vi "SetNumber.vi"(6 "i":i32, 7 "Agentes Disponíveis":dbl, 10 "Used numbers":dbl[](array[numeric]), 11 "element":T1={"id"=0, "function"=enum."Attacker", "x"=0.0, "y"=0.0, "orientation"=0.0, "v_tangent"=0.0, "v_normal"=0.0, "v_ang"=0.0, "kick_x"=0.0, "kick_z"=0.0, "dribble"=FALSE, "Timestamp"=timestamp(0 s since 1904-01-01), "estimatives"={"est_v_tangent"=0.0, "est_v_normal"=0.0, "est_vx"=0.0, "est_vy"=0.0, "Pos Robot Est"=[]}, "dest_x_kick"=0.0, "dest_y_kick"=0.0, "Gap Coord"=[], "States"=enum."GoToTangent", "Path "=[], "Path  Smooth"=[], "Dest"=[], "Missões "=enum."Monitorar Comboio", "Agentes Disponíveis"=0.0, "Number"=0.0} {"Agentes Disponíveis" format="%#_13g"}) -> (0 "i out":i32, 3 "element out":T1={"id"=0, "function"=enum."Attacker", "x"=0.0, "y"=0.0, "orientation"=0.0, "v_tangent"=0.0, "v_normal"=0.0, "v_ang"=0.0, "kick_x"=0.0, "kick_z"=0.0, "dribble"=FALSE, "Timestamp"=timestamp(0 s since 1904-01-01), "estimatives"={"est_v_tangent"=0.0, "est_v_normal"=0.0, "est_vx"=0.0, "est_vy"=0.0, "Pos Robot Est"=[]}, "dest_x_kick"=0.0, "dest_y_kick"=0.0, "Gap Coord"=[], "States"=enum."GoToTangent", "Path "=[], "Path  Smooth"=[], "Dest"=[], "Missões "=enum."Monitorar Comboio", "Agentes Disponíveis"=0.0, "Number"=0.0} {"Agentes Disponíveis" format="%#_13g"})   [LabVIEW 2018]
uses:
  Core/AI Robot.ctl
  Intel/Functions Enum.ctl
  Intel/AttackerStates.ctl
  Path Planning/RRT/PathDests.ctl
  Path Planning/RRT/PathDest.ctl
panel:
  out "Array 2":dbl[](array[numeric])
  out "unused numbers":dbl[](array[numeric])
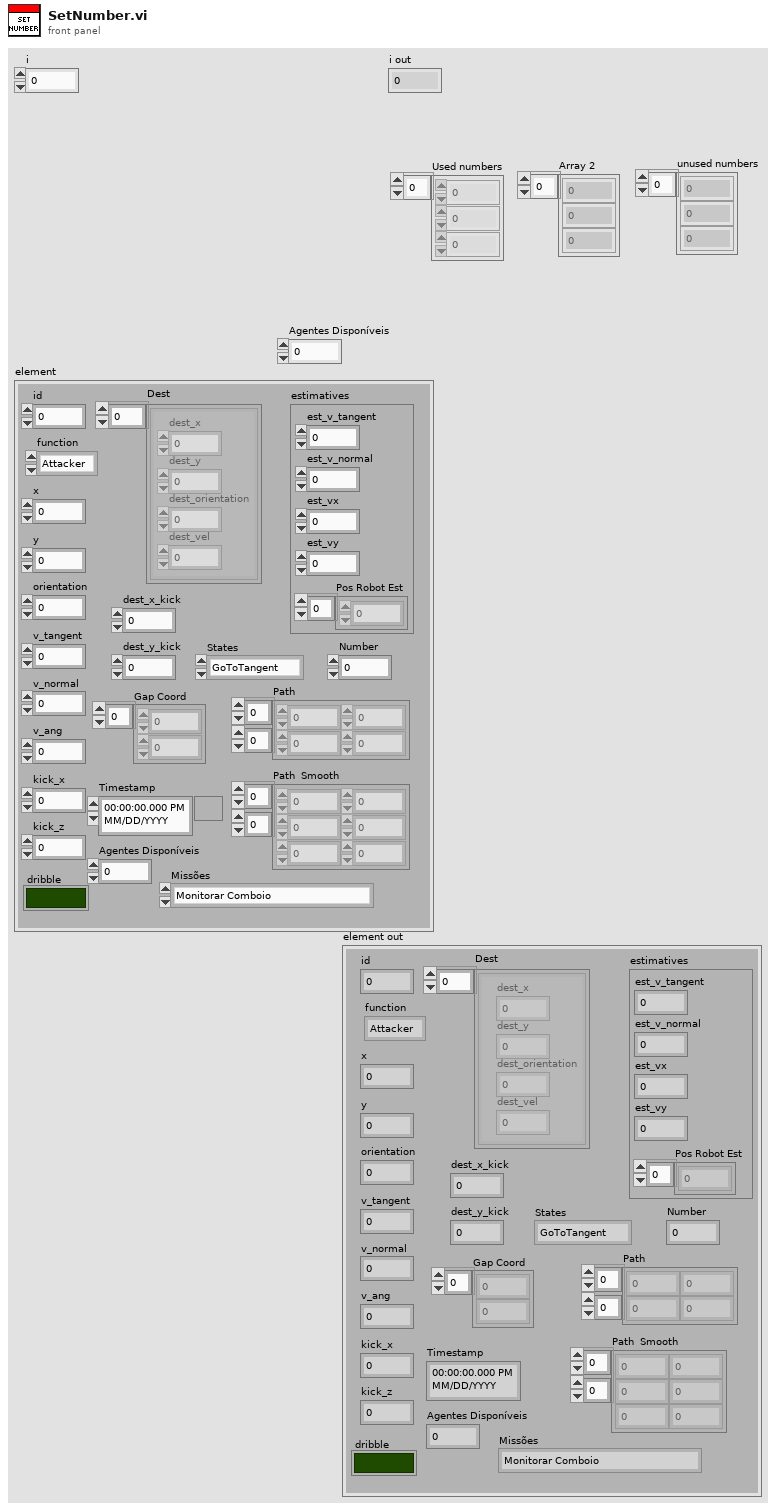
[diagram p1: front panel]
types:
  T1 = typedef "AI Robot.ctl" = cluster{"id":u32, "function":T2, "x":dbl, "y":dbl, "orientation":dbl, "v_tangent":dbl, "v_normal":dbl, "v_ang":dbl, "kick_x":dbl, "kick_z":dbl, "dribble":bool, "Timestamp":timestamp, "estimatives":cluster{"est_v_tangent":dbl, "est_v_normal":dbl, "est_vx":dbl, "est_vy":dbl, "Pos Robot Est":dbl[]}, "dest_x_kick":dbl, "dest_y_kick":dbl, "Gap Coord":dbl[], "States":T3, "Path ":dbl[][], "Path  Smooth":dbl[][], "Dest":T4, "Missões ":enum16{"Monitorar Comboio", "Realizar Segurança de Retaguarda", "Vigiar Área", "Reconhecimento de Área"}, "Agentes Disponíveis":dbl, "Number":dbl}
  T2 = typedef "Functions Enum.ctl" = enum16{"None", "Vigia", "2nd Striker", "Attacker", "Goalie", "Defender", "Striker", "Goto 0", "Dummy", "Kicker", "ZigZag 0", "ZigZag 1", "ZigZag 2", "ZigZag 3", "ZigZag 4", "ZigZag 5", "ZigZag 6", "ZigZag 7", "ZigZag 8", ""}
  T3 = typedef "AttackerStates.ctl" = enum16{"Pass", "GoToTangent", "BallGetting", "GoToKick", ""}
  T4 = typedef "PathDests.ctl" = T5[]
  T5 = typedef "PathDest.ctl" = cluster{"dest_x":dbl, "dest_y":dbl, "dest_orientation":dbl, "dest_vel":dbl}
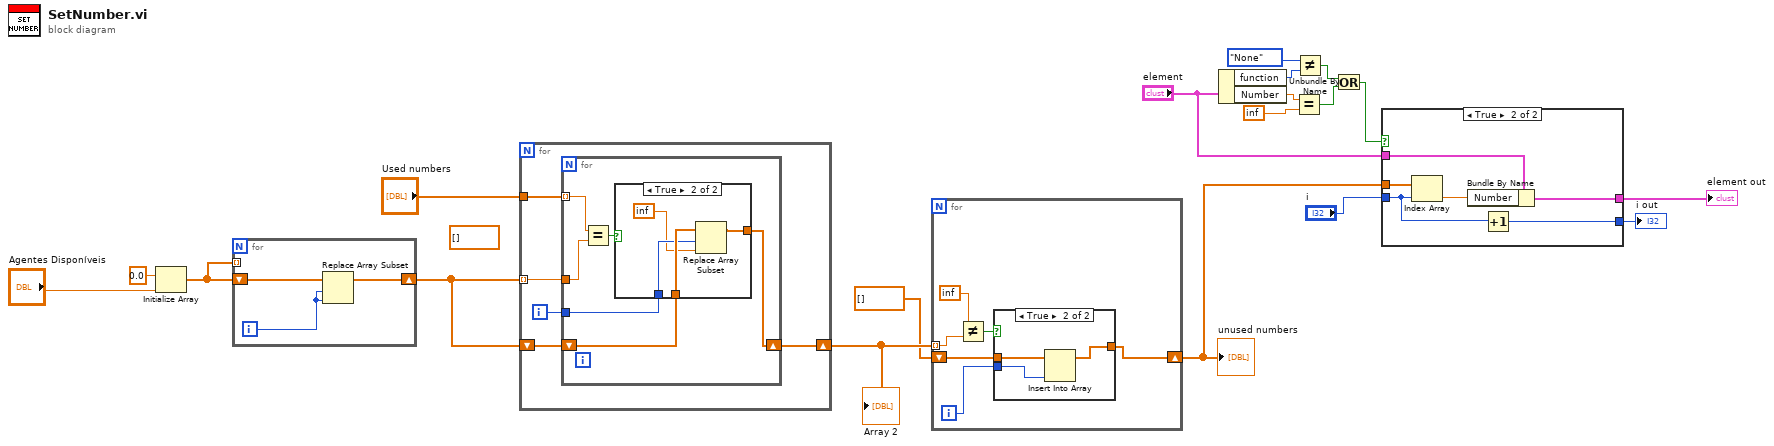
[diagram p0: block diagram]
diagram:
  (unwired) dbl[] []
  n1 = Initialize Array(0.0 ("element"), "Agentes Disponíveis") -> (w19:dbl[])
  n2 = for {
    tunnel: w19 -> [_] mode=indexing
    shift-right: [w20] -> w15
    shift-left: w19 -> [w22]
    i -> [w21]
    n3 = Replace Array Subset(array=w22, new element=w21, index=w21) -> (w20:dbl[])
  }
  n4 = for {
    tunnel: "Used numbers" -> [w27]
    tunnel: w15 -> [w26] mode=indexing
    shift-right: [w23] -> w14
    shift-left: w15 -> [w24]
    i -> [w25]
    n5 = for {
      tunnel: w27 -> [w32] mode=indexing
      tunnel: w26 -> [w31]
      tunnel: w25 -> [w30]
      shift-right: [w28] -> w23
      shift-left: w24 -> [w29]
      n6 = Equal?(x=w32, y=w31) -> (x = y?=w33:bool)
      n7 = case shown="True" w33 {
        tunnel: w30 -> [_ w36]
        tunnel: [w34 w38] -> w28
        tunnel: w29 -> [w34 w37]
        frame False {
        }
        frame True {
          n8 = Replace Array Subset(array=w37, new element=inf, index=w36) -> (w38:dbl[])
        }
      }
    }
  }
  "Array 2" <- w14
  n9 = for {
    tunnel: w14 -> [w44] mode=indexing
    shift-right: [w39] -> w4
    shift-left: dbl[] [] -> [w40]
    i -> [w41]
    n10 = Not Equal?(x=inf, y=w44) -> (x != y?=w43:bool)
    n11 = case shown="True" w43 {
      tunnel: w41 -> [_ w48]
      tunnel: w40 -> [w45 w47]
      tunnel: [w45 w46] -> w39
      frame False {
      }
      frame True {
        n12 = Insert Into Array(array=w47, new element=w48) -> (w46:dbl[])  [unwired: 1 in]
      }
    }
  }
  "unused numbers" <- w4
  n13 = Unbundle By Name("element") -> ("function"=w11:T2, "Number"=w12:dbl)
  n14 = Equal?(x=w12, y=inf) -> (x = y?=w7:bool)
  n15 = Not Equal?(x=Functions_Enum."None", y=w11) -> (x != y?=w8:bool)
  n16 = Or(x=w8, y=w7) -> (x .or. y?=w6:bool)
  n17 = case shown="True" w6 {
    tunnel: "element" -> [w50 w56]
    tunnel: w4 -> [_ w55]
    tunnel: "i" -> [w49 w52]
    tunnel: [w50 w53] -> w2
    tunnel: [w49 w51] -> w1
    frame False {
    }
    frame True {
      n18 = Index Array(array=w55, index=w52) -> (element=w54:dbl)
      n19 = Bundle By Name(cluster=w56, "Number"=w54) -> (w53:T1)
      n20 = Increment(x=w52) -> (x+1=w51:i32)
    }
  }
  "element out" <- w2
  "i out" <- w1
